vi "SRingBlockTrig_SD.vi"(1 "channel 1, 2 or 3":u8=1) -> (0 "Boolesch":bool)   [LabVIEW 2015]
uses:
  DLL/ESLSCDLL.dll
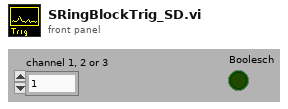
[diagram p1: front panel]
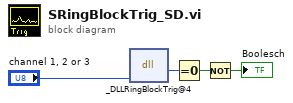
[diagram p0: block diagram]
diagram:
  n1 = dll-call lib="G:/SD/TRANCON/DLL/ESLSCDLL.dll" fn="_DLLRingBlockTrig@4" ("lwlscdll.dll:DLLTempGood")("ch"="channel 1, 2 or 3") -> ("Rückgabetyp"=w3:u8)  [unwired: 4 in, 2 out]
  n2 = Equal To 0?(x=w3) -> (x = 0?=w2:bool)
  n3 = Not(x=w2) -> (.not. x?=→"Boolesch":bool)
